vi "get-Position-v2.vi"(8 "error in (no error)":errorcluster) -> (0 "error out":errorcluster, 1 "Position Z":sgl, 2 "Position Y":dbl, 3 "Position X":dbl)   [LabVIEW 2014]
doc: "André Romero - 2023\nandretec@ifsc.usp.br\nIFSC - USP"
uses:
  Global Motors.vi
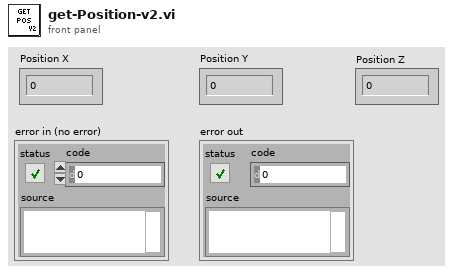
[diagram p1: front panel]
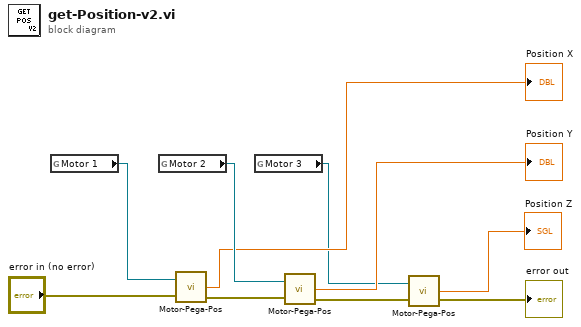
[diagram p0: block diagram]
diagram:
  n1 = global read "Global Motors.vi" "Motor 1"() -> (w8:refnum<k7>)
  n2 = global read "Global Motors.vi" "Motor 2"() -> (w7:refnum<k7>)
  n3 = call "Motor-Pega-Pos.vi"("MG17Motor 2"=w8, "error out"="error in (no error)") -> ("pfPosition"=→"Position X":sgl, "error out 2"=w9:errorcluster)  [unwired: 1 out]
  n4 = global read "Global Motors.vi" "Motor 3"() -> (w3:refnum<k7>)
  n5 = call "Motor-Pega-Pos.vi"("MG17Motor 2"=w7, "error out"=w9) -> ("pfPosition"=→"Position Y":sgl, "error out 2"=w4:errorcluster)  [unwired: 1 out]
  n6 = call "Motor-Pega-Pos.vi"("MG17Motor 2"=w3, "error out"=w4) -> ("pfPosition"=→"Position Z":sgl, "error out 2"=→"error out":errorcluster)  [unwired: 1 out]
